vi "include.get.vi"(8 "error in (no error)":errorcluster, 11 "include in":refnum<class "include.lvclass">) -> (0 "error out":errorcluster, 2 "include":set{refnum<class "filterTypes.lvclass">}(c389), 3 "include out":refnum<class "include.lvclass">)   [LabVIEW 2020, in "nominal types.lvlib" / "channelFilter.lvlib" / "include.lvclass"]
uses:
  include.lvclass
  include.lvclass/include.ctl
  filterTypes/filterTypes.lvclass
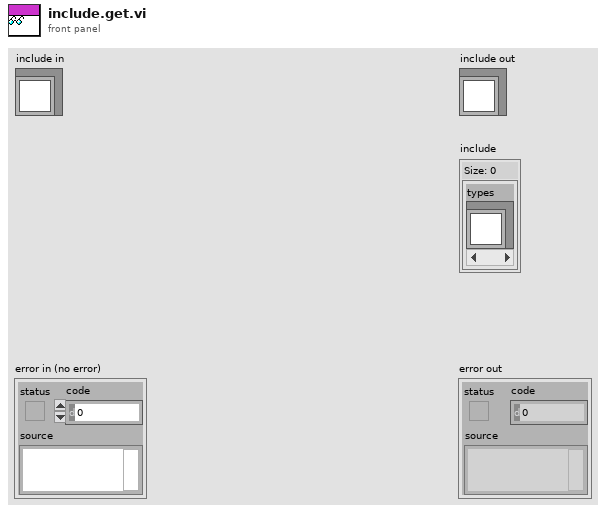
[diagram p1: front panel]
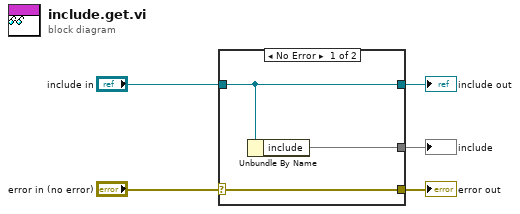
[diagram p0: block diagram]
diagram:
  n1 = case shown="No Error" "error in (no error)" {
    selector: "error in (no error)" -> [w6 w9]
    tunnel: [w6 w9] -> w4
    tunnel: [w8 w10] -> w2
    tunnel: "include in" -> [w8 w10]
    tunnel: [w7 _] -> w1
    frame No Error {
      n2 = Unbundle By Name(w8) -> ("include"=w7:set{refnum<class "filterTypes.lvclass">})
    }
    frame Error {
    }
  }
  "error out" <- w4
  "include out" <- w2
  "include" <- w1
